vi "Read Temperature.vi"(8 "error in":errorcluster, 10 "SI":T1, 11 "TC01 in":refnum<class "TC01.lvclass">) -> (0 "error out":errorcluster, 2 "Temperature":dbl, 3 "TC01 out":refnum<class "TC01.lvclass">)   [LabVIEW 2018, in "TC01.lvlib" / "TC01.lvclass"]
uses:
  TC01.lvclass
  PPLs/Thermocouple/Thermocouple.lvlibp/Custom Controls/System Units.ctl
  TC01.lvclass/TC01.ctl
  <vilib>/DAQmx/read.llb/DAQmx Read (Analog DBL 1Chan 1Samp).vi
  <vilib>/DAQmx/miscellaneous.llb/DAQmx Fill In Error Info.vi
  PPLs/Thermocouple/Thermocouple.lvlibp
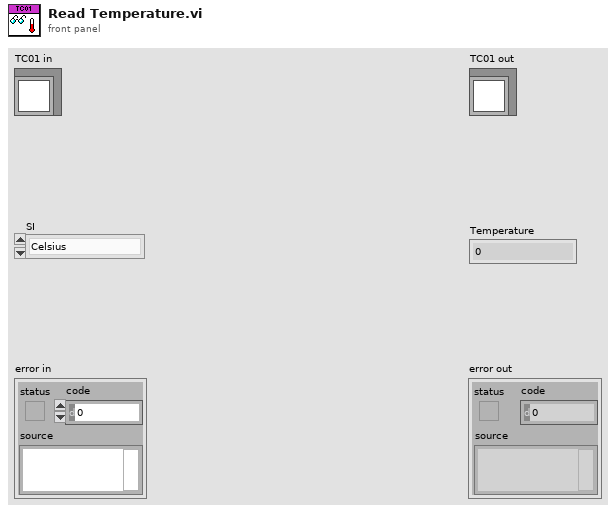
[diagram p1: front panel]
types:
  T1 = typedef "Thermocouple.lvlibp/System Units.ctl" = enum16{"Celsius", "Fahrenheit"}
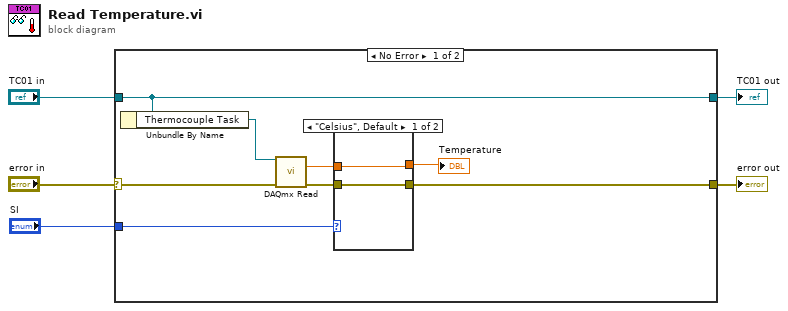
[diagram p0: block diagram]
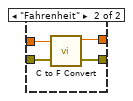
[diagram p2: hidden frame]
diagram:
  n1 = case shown="No Error" "error in" {
    selector: "error in" -> [w13 w20]
    tunnel: [w9 w20] -> w4
    tunnel: "TC01 in" -> [w11 w19]
    tunnel: [w11 w19] -> w2
    tunnel: "SI" -> [w7 _]
    frame No Error {
      n2 = Unbundle By Name(w11) -> ("Thermocouple Task"=w12:refnum<k21>)
      n3 = call-poly <vilib>:"DAQmx Read.vi"("task/channels in"=w12, "error in"=w13) -> ("data"=w8:dbl, "error out"=w10:errorcluster)  [unwired: 11 in, 1 out]
      n4 = case shown="\"Celsius\", Default" w7 {
        tunnel: w10 -> [w15 w18]
        tunnel: [w15 w18] -> w9
        tunnel: w8 -> [w14 w17]
        tunnel: [w14 w16] -> w6
        frame "Celsius", Default {
        }
        frame "Fahrenheit" {
          n5 = call "C to F Convert.vi"("°C"=w17) -> ("°F"=w16:dbl)  [unwired: 10 in]
        }
      }
      "Temperature" <- w6
    }
    frame Error {
    }
  }
  "error out" <- w4
  "TC01 out" <- w2
